vi "Untitled 4.vi"(1 "data":dynamicdata(waveform), 4 "timeout (s)":dbl=10.0 format="%0.2f", 5 "error in":errorcluster, 7 "stop (T)":bool=TRUE, 10 "device name":tag="Dev1") -> (14 "task out":refnum<k21>, 19 "error out":errorcluster)   [LabVIEW 2017]
doc: "Creates, edits, and runs tasks using NI-DAQmx. Refer to the NI-DAQmx Readme for a complete listing of devices NI-DAQmx supports.\n\nWhen you place this Express VI on the block diagram, the DAQ Assistant launches to create a new task. After you create a task, you can double-click the DAQ Assistant Express VI to edit that task. For continuous measurement or generation, place a while loop around the DAQ Assistant Express VI."
uses:
  <vilib>/DAQmx/write.llb/DAQmx Write.vi
  <vilib>/DAQmx/write.llb/DAQmx Write (Analog 1D Wfm NChan NSamp).vi
  <vilib>/DAQmx/miscellaneous.llb/DAQmx Fill In Error Info.vi
  <vilib>/DAQmx/configure/timing.llb/DAQmx Timing (Use Waveform).vi
  <vilib>/DAQmx/configure/timing.llb/DAQmx Timing (Sample Clock).vi
  <vilib>/DAQmx/create/channels.llb/DAQmx Create Channel (AO-Voltage-Basic).vi
  <resource>/objmgr/daqmx.rc
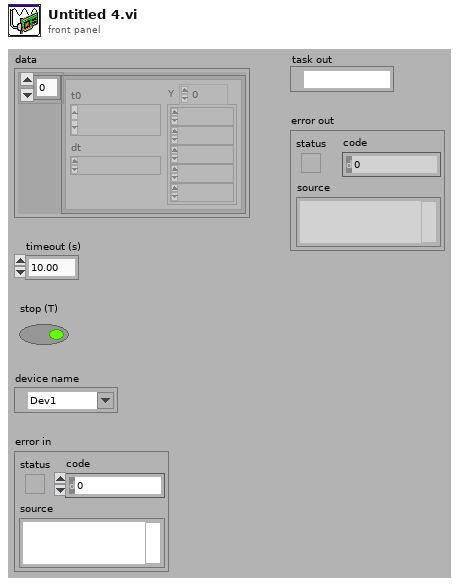
[diagram p1: front panel]
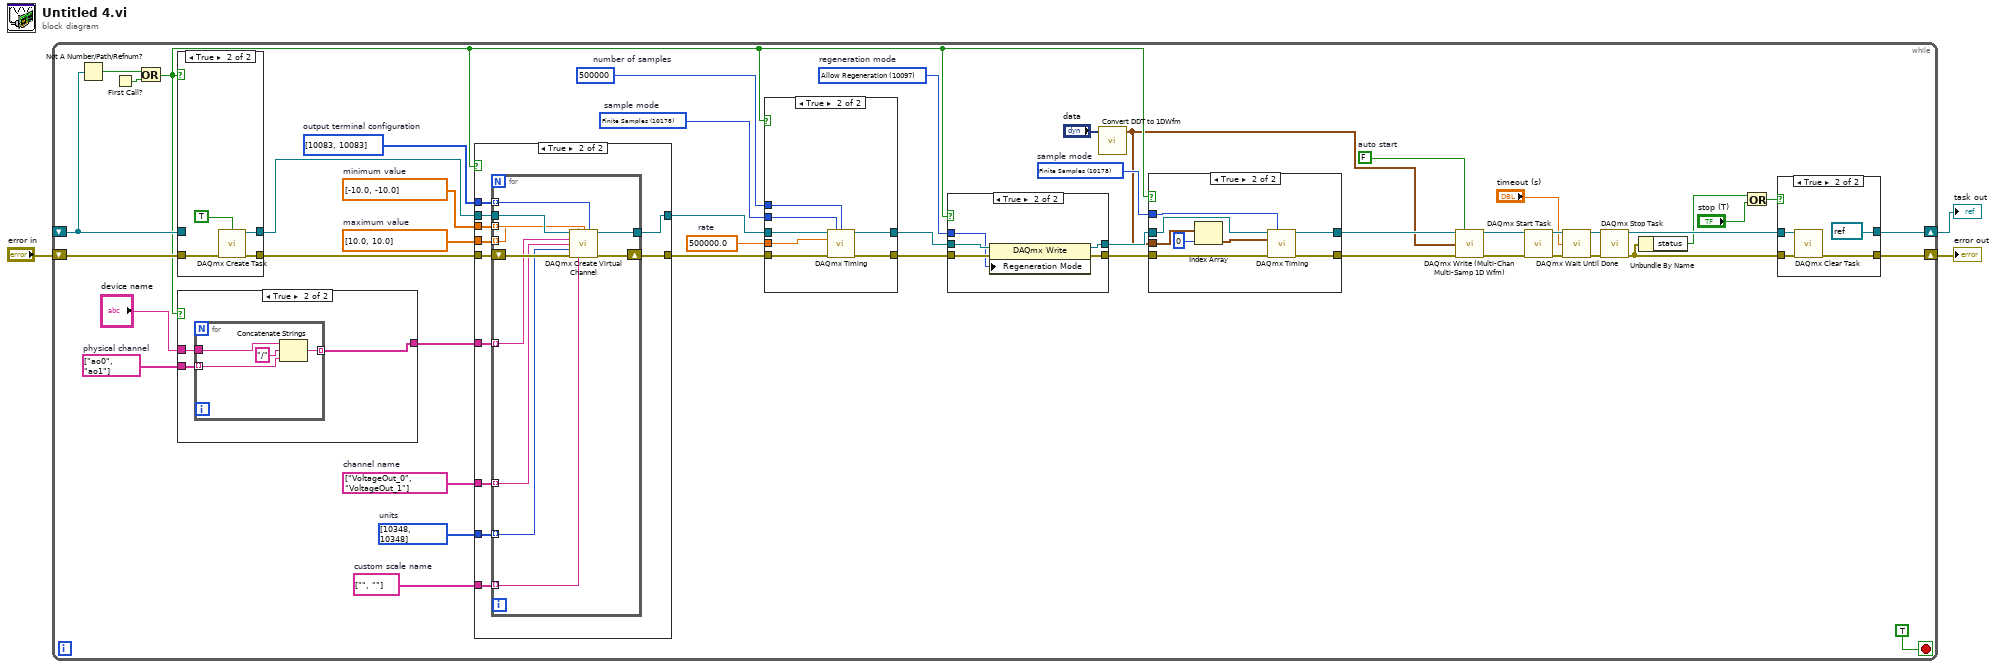
[diagram p0: block diagram]
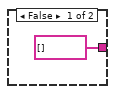
[diagram p7: hidden frame]
diagram:
  n1 = while {
    shift-right: [w10] -> w1
    shift-left: _ -> [w47]
    shift-right: [w4] -> w2
    shift-left: "error in" -> [w48]
    stop <- TRUE stop-if-true
    w23 = 10178 items=["Finite Samples"=10178, "Continuous Samples"=10123]  # sample mode
    w26 = FALSE  # auto start
    w27 = 10097 items=["Allow Regeneration"=10097, "Do Not Allow Regeneration"=10158]  # regeneration mode
    w30 = 10178 items=["Finite Samples"=10178, "Continuous Samples"=10123, "Hardware Timed Single Point"=12522]  # sample mode
    w31 = 500000.0  # rate
    w32 = 500000  # number of samples
    w35 = i32[] [10083, 10083] items=["Default"=-1, "RSE"=10083, "Differential"=10106, "Pseudodifferential"=12529]  # output terminal configuration
    w36 = string[] ["", ""]  # custom scale name
    w37 = i32[] [10348, 10348] items=["Volts"=10348, "From Custom Scale"=10065]  # units
    w38 = string[] ["VoltageOut_0", "VoltageOut_1"]  # channel name
    w40 = dbl[] [10.0, 10.0]  # maximum value
    w41 = dbl[] [-10.0, -10.0]  # minimum value
    w44 = string[] ["ao0", "ao1"]  # physical channel
    n2 = Not A Number/Path/Refnum?(number/path/refnum=w47) -> (NaN/Path/Refnum?=w46:bool)
    n3 = First Call?() -> (First Call?: T/F=w49:bool)
    n4 = Or(x=w46, y=w49) -> (x .or. y?=w24:bool)
    n5 = case shown="True" w24 {
      tunnel: [w116 w120] -> w43
      tunnel: w47 -> [w116 _]
      tunnel: [w115 w119] -> w42
      tunnel: w48 -> [w115 w117]
      frame False {
      }
      frame True {
        n6 = call <vilib>:"DAQmx Create Task.vi"("auto cleanup"=TRUE, "error in"=w117) -> ("task out"=w120:refnum<k21>, "error out"=w119:errorcluster)  [unwired: 12 in]
      }
    }
    n7 = case shown="True" w24 {
      tunnel: [string[] [] w110] -> w39
      tunnel: "device name" -> [_ w109]
      tunnel: w44 -> [_ w108]
      frame False {
      }
      frame True {
        n8 = for {
          tunnel: [w114] -> w110 mode=indexing
          tunnel: w109 -> [w113]
          tunnel: w108 -> [w111] mode=indexing
          n9 = Concatenate Strings(w113, "/" ("string"), w111) -> (w114:string)
        }
      }
    }
    n10 = case shown="True" w24 {
      tunnel: [w84 w93] -> w34
      tunnel: w43 -> [w84 w95]
      tunnel: [w83 w92] -> w33
      tunnel: w42 -> [w83 w94]
      tunnel: w41 -> [_ w91]
      tunnel: w40 -> [_ w90]
      tunnel: w39 -> [_ w89]
      tunnel: w38 -> [_ w88]
      tunnel: w37 -> [_ w87]
      tunnel: w36 -> [_ w86]
      tunnel: w35 -> [_ w85]
      frame False {
      }
      frame True {
        n11 = for {
          tunnel: w95 -> [w106]
          tunnel: [w104] -> w93
          tunnel: w91 -> [w102] mode=indexing
          tunnel: w90 -> [w101] mode=indexing
          tunnel: w89 -> [w100] mode=indexing
          tunnel: w88 -> [w99] mode=indexing
          tunnel: w87 -> [w98] mode=indexing
          tunnel: w86 -> [w97] mode=indexing
          shift-right: [w103] -> w92
          shift-left: w94 -> [w105]
          tunnel: w85 -> [w96] mode=indexing
          n12 = call-poly <vilib>:"DAQmx Create Virtual Channel.vi"("task in"=w106, "maximum value"=w101, "minimum value"=w102, "output terminal configuration"=w96, "physical channels"=w100, "name to assign"=w99, "units"=w98, "error in"=w105, "custom scale name"=w97) -> ("task out"=w104:refnum<k21>, "error out"=w103:errorcluster)  [unwired: 5 in]
        }
      }
    }
    n13 = case shown="True" w24 {
      tunnel: [w75 w77] -> w29
      tunnel: w34 -> [w75 w80]
      tunnel: [w74 w76] -> w28
      tunnel: w33 -> [w74 w78]
      tunnel: w32 -> [_ w82]
      tunnel: w30 -> [_ w81]
      tunnel: w31 -> [_ w79]
      frame False {
      }
      frame True {
        n14 = call-poly <vilib>:"DAQmx Timing.vi"("task/channels in"=w80, "sample mode"=w81, "samples per channel"=w82, "rate"=w79, "error in"=w78) -> ("task out"=w77:refnum<k21>, "error out"=w76:errorcluster)  [unwired: 9 in]
      }
    }
    n15 = case shown="True" w24 {
      tunnel: w29 -> [w68 w73]
      tunnel: [w68 w72] -> w19
      tunnel: w28 -> [w67 w71]
      tunnel: [w67 w70] -> w20
      tunnel: w27 -> [_ w69]
      frame False {
      }
      frame True {
        n16 = property class="DAQmx Write"(reference=w73, error in=w71, "Regeneration Mode"=w69) -> (reference out=w72:refnum<k21>, error out=w70:errorcluster)
      }
    }
    n17 = call <vilib>:"Convert DDT to 1DWfm.vi"("Dynamic Data Type"="data") -> ("Array of Waveforms"=w18:waveform(dbl)[])  [unwired: 3 in]
    n18 = case shown="True" w24 {
      tunnel: [w58 w63] -> w22
      tunnel: w19 -> [w58 w65]
      tunnel: [w57 w62] -> w21
      tunnel: w20 -> [w57 w64]
      tunnel: w23 -> [_ w66]
      tunnel: w18 -> [_ w60]
      frame False {
      }
      frame True {
        n19 = Index Array(array=w60, index=0) -> (element=w59:waveform(dbl))
        n20 = call-poly <vilib>:"DAQmx Timing.vi"("task/channels in"=w65, "sample mode"=w66, "waveform"=w59, "error in"=w64) -> ("task out"=w63:refnum<k21>, "error out"=w62:errorcluster)  [unwired: 10 in]
      }
    }
    n21 = call-poly "DAQmx Write (Multi-Chan Multi-Samp 1D Wfm).vi"("task/channels in"=w22, "auto start"=w26, "data"=w18, "error in"=w21) -> ("task out"=w13:refnum<k21>, "error out"=w12:errorcluster)  [unwired: 9 in, 1 out]
    n22 = call <vilib>:"DAQmx Start Task.vi"("task/channels in"=w13, "error in"=w12) -> ("task out"=w17:refnum<k21>, "error out"=w16:errorcluster)  [unwired: 12 in]
    n23 = call <vilib>:"DAQmx Wait Until Done.vi"("task/channels in"=w17, "timeout (sec)"="timeout (s)", "error in"=w16) -> ("task out"=w14:refnum<k21>, "error out"=w15:errorcluster)  [unwired: 11 in]
    n24 = call <vilib>:"DAQmx Stop Task.vi"("task/channels in"=w14, "error in"=w15) -> ("task out"=w11:refnum<k21>, "error out"=w8:errorcluster)  [unwired: 12 in]
    n25 = Unbundle By Name(w8) -> ("status"=w7:bool)
    n26 = Or(x=w7, y="stop (T)") -> (x .or. y?=w5:bool)
    n27 = case shown="True" w5 {
      tunnel: w11 -> [w52 w56]
      tunnel: [w52 refnum<k21> refnum ("task in")] -> w10
      tunnel: w8 -> [w51 w55]
      tunnel: [w51 w54] -> w4
      frame False {
      }
      frame True {
        n28 = call <vilib>:"DAQmx Clear Task.vi"("task in"=w56, "error in"=w55) -> ("error out"=w54:errorcluster)  [unwired: 13 in]
      }
    }
  }
  "error out" <- w2
  "task out" <- w1
